vi "GetDefaultParams.vi"(8 "error in (no error)":errorcluster, 10 "config file path":path, 11 "Class In":refnum<class "NiPxi6733.lvclass">) -> (0 "error out":errorcluster, 3 "Class Out":refnum<class "NiPxi6733.lvclass">)   [LabVIEW 2014, in "FGenPlugins.lvlib" / "NiPxi6733.lvclass"]
uses:
  NiPxi6733.lvclass
  TypeDefs/clTimebase.ctl
  <userlib>/NIST/BaseClasses/BasePlugin_class/BasePlugin.lvclass/BasePlugin.ctl
  NiPxi6733.lvclass/NiPxi6733.ctl
  <userlib>/NIST/BaseClasses/BasePlugin_class/Accessors/Read PluginIniFilePath.vi
  Accessors/Write Timebase.vi
  NiBaseClass/NiBase.lvclass
  <vilib>/Utility/config.llb/NI_LVConfig.lvlib
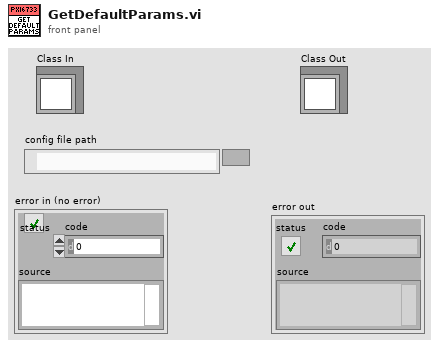
[diagram p1: front panel]
types:
  T1 = typedef "FGenPlugins.lvlib/NiPxi6733.lvclass/clTimebase.ctl" = cluster{"Src":tag, "Rate":dbl}
  T2 = typedef "NI_LVConfig.lvlib/Config Data RefNum.ctl" = refnum<k1>
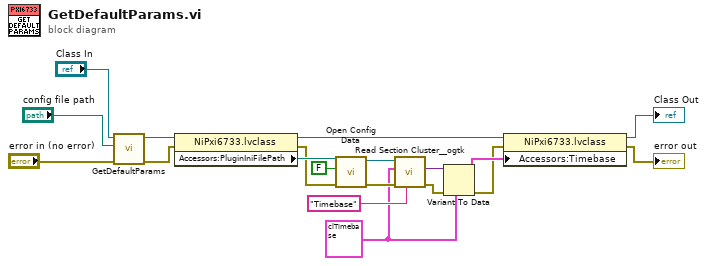
[diagram p0: block diagram]
diagram:
  w5 = T1 {"Src"="/PXI1Slot6/PXI_Star", "Rate"=20000000.0} ("clTimebase")
  n1 = call-parent "GetDefaultParams.vi"("error in (no error)"="error in (no error)", "config file path"="config file path", "Class In"="Class In") -> ("error out"=w14:errorcluster, "Class Out"=w19:refnum<class "NiPxi6733.lvclass">)  [unwired: 7 in]
  n2 = property class="NiPxi6733.lvclass"(reference=w19, error in=w14) -> (reference out=w15:refnum<class "NiPxi6733.lvclass">, error out=w12:errorcluster, "Accessors:PluginIniFilePath"=w13:path)
  n3 = call <vilib>:"Open Config Data.vi"("error in (no error)"=w12, "create file if necessary (T)"=FALSE, "configuration file path"=w13) -> ("error out"=w10:errorcluster, "refnum"=w9:T2)  [unwired: 6 in, 1 out]
  n4 = call <userlib>:"Read Section Cluster__ogtk.vi"("section (optional)"="Timebase", "error in (no error)"=w10, "Section Formatted Cluster Type"=w5, "refnum"=w9) -> ("error out"=w6:errorcluster, "Section Formatted Cluster"=w7:variant)  [unwired: 3 in, 3 out]
  n5 = Variant To Data(error in=w6, type=w5, Variant=w7) -> (data=w3:T1, error out=w2:errorcluster)
  n6 = property class="NiPxi6733.lvclass"(reference=w15, error in=w2, "Accessors:Timebase"=w3) -> (reference out=→"Class Out":refnum<class "NiPxi6733.lvclass">, error out=→"error out":errorcluster)
